vi "Index Based on Type.vi"(8 "Error In":errorcluster, 10 "Type code Array":i32[](array[numeric])) -> (0 "Error Out":errorcluster, 1 "2D array Index":u32[](array[numeric]), 2 "1D array Index":u32[](array[numeric]), 3 "Scalar Index":u32[](array[numeric]), 5 "Type code Array dup":i32[](array[numeric]))   [LabVIEW 2014]
doc: "<B>Copyright</B>: (c) MHWirth 2015.\n\nThis VI generates 3 arrays which contain the indeces for scalars, 1D arrays, and 2D arrays based on the input <B>Type code Array</B>. \n\n<B>Error 7001</B>: Unknown Data Type - Type Code Array (Int32) contains -1 indicating an unknown data type."
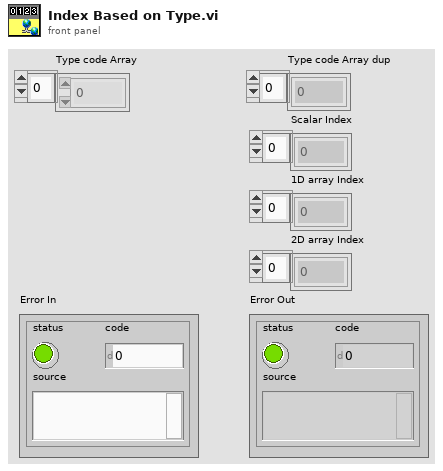
[diagram p1: front panel]
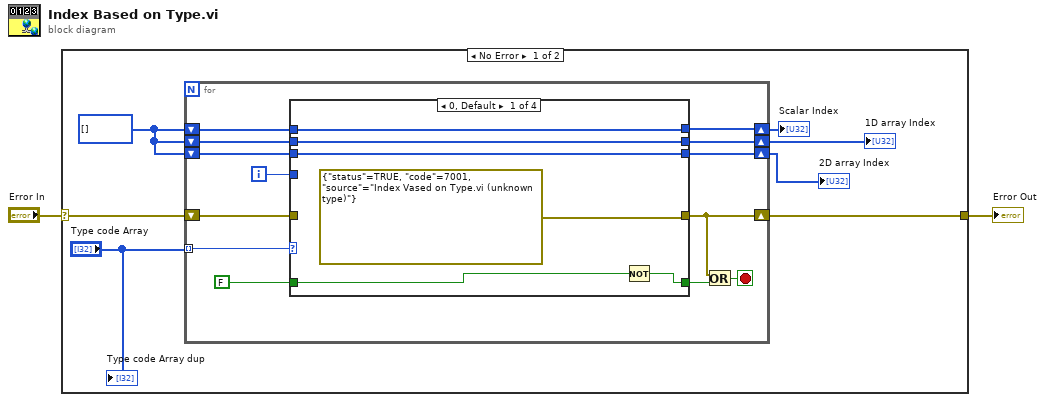
[diagram p0: block diagram]
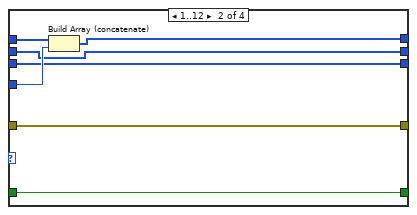
[diagram p2: hidden frame]
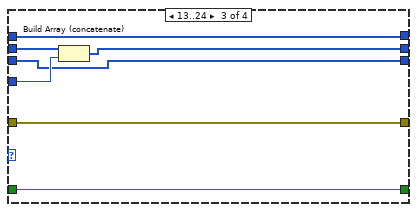
[diagram p3: hidden frame]
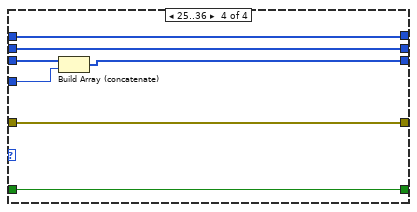
[diagram p4: hidden frame]
diagram:
  n1 = case shown="No Error" "Error In" {
    selector: "Error In" -> [w9 w50]
    tunnel: [w8 w50] -> w1
    frame No Error {
      w6 = u32[] []
      n2 = for {
        shift-right: [w18] -> w8
        shift-left: w9 -> [w20]
        tunnel: "Type code Array" -> [w21] mode=indexing
        shift-right: [w15] -> w5
        shift-left: w6 -> [w17]
        shift-right: [w11] -> w4
        shift-left: w6 -> [w13]
        shift-right: [w10] -> w3
        shift-left: w6 -> [w12]
        i -> [w14]
        stop <- w19 stop-if-true
        n3 = case shown="0, Default" w21 {
          tunnel: FALSE -> [w27 w34 w40 w47]
          tunnel: w20 -> [_ w35 w42 w49]
          tunnel: [errorcluster {"status"=TRUE, "code"=7001, "source"="Index Vased on Type.vi (unknown type)"} ("error constant") w35 w42 w49] -> w18
          tunnel: w17 -> [w25 w33 w41 w48]
          tunnel: [w26 w34 w40 w47] -> w16
          tunnel: [w25 w31 w41 w48] -> w15
          tunnel: w13 -> [w24 w29 w39 w43]
          tunnel: w12 -> [w23 w30 w37 w45]
          tunnel: w14 -> [_ w32 w38 w46]
          tunnel: [w24 w29 w36 w43] -> w11
          tunnel: [w23 w30 w37 w44] -> w10
          frame 0, Default {
            n4 = Not(x=w27) -> (.not. x?=w26:bool)
          }
          frame 1..12 {
            n5 = Build Array (concatenate)(w33, w32) -> (w31:u32[])
          }
          frame 13..24 {
            n6 = Build Array (concatenate)(w39, w38) -> (w36:u32[])
          }
          frame 25..36 {
            n7 = Build Array (concatenate)(w45, w46) -> (w44:u32[])
          }
        }
        n8 = Or(x=w18, y=w16) -> (x .or. y?=w19:bool)
      }
      "Scalar Index" <- w5
      "1D array Index" <- w4
      "2D array Index" <- w3
      "Type code Array dup" <- "Type code Array"
    }
    frame Error {
    }
  }
  "Error Out" <- w1
